vi "UnRegisterWithNode.vi"(0 "ROS":T3={"topic port"=0, "Node"="", "topic"="", "type"="", "node port"=0, "error "={"status"=FALSE, "code"=0, "source"=""}, "Direction"=enum."Node", "APIs"=[], "Update (ms)"=1, "write queue"=1}, 1 "Err in":string) -> (2 "MyState":T2, 3 "Log":T1, 4 "Err out":string)   [LabVIEW 2010]
uses:
  SubVIs/_ROSDirection.ctl
  SubVIs/_ROSControl.ctl
  ROSLog.ctl
  MyState.ctl
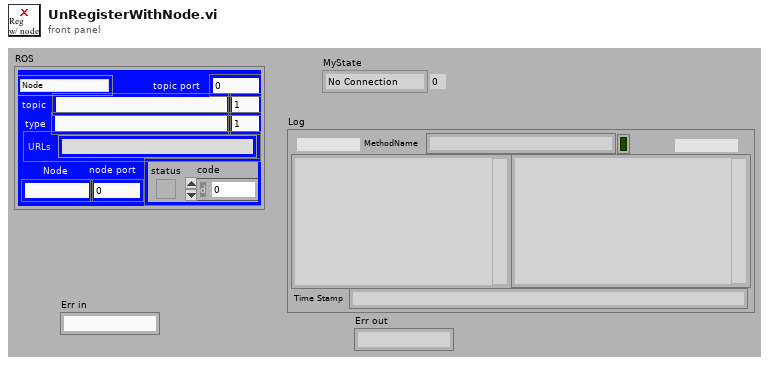
[diagram p1: front panel]
types:
  T1 = typedef "ROSLog.ctl" = cluster{"Sent":string, "Reply":string, "MethodName":string, "success":bool, "Dir1":string, "Dir2":string, "Time Stamp":string}
  T2 = typedef "MyState.ctl" = enum16{"No Connection", "Registered", "Connected", "Close"}
  T3 = typedef "_ROSControl.ctl" = cluster{"topic port":u16, "Node":string, "topic":string, "type":string, "node port":u32, "error ":errorcluster, "Direction":T4, "APIs":string[], "Update (ms)":u16, "write queue":u16}
  T4 = typedef "_ROSDirection.ctl" = enum16{"Node", "Publisher", "Subscriber", "Service Client"}
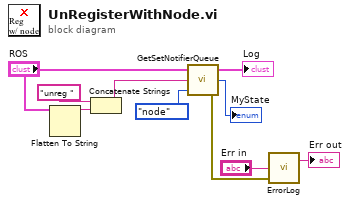
[diagram p0: block diagram]
diagram:
  n1 = Flatten To String(anything="ROS") -> (data string=w8:string)  [unwired: 3 in, 2 out]
  n2 = Concatenate Strings("unreg " ("element"), w8) -> (w6:string)
  n3 = call "GetSetNotifierQueue.vi"("Name"=enum16{"topic", "node"}."node", "Command"=w6, "ROS"="ROS") -> ("error out"=w3:errorcluster, "MyState"=→"MyState":T2, "Log"=→"Log":T1)
  n4 = call "ErrorLog.vi"("error in"=w3, "String in"="Err in") -> ("String out"=→"Err out":string)  [unwired: 1 in, 1 out]
